vi "Read configuration.vi"(8 "error in":errorcluster, 11 "ExampleSequencer editor node in":refnum<class "ExampleSequencer editor node.lvclass">) -> (0 "error out":errorcluster, 2 "configuration":refnum<class "NISE_CEF_serializable configuration.lvclass">, 3 "ExampleSequencer editor node out":refnum<class "ExampleSequencer editor node.lvclass">)   [LabVIEW 2017, in "ExampleSequencer editor node.lvclass"]
uses:
  ExampleSequencer editor node.lvclass
  <vilib>/NI/Configuration Framework/serializable configuration/NISE_CEF_serializable configuration.lvclass
  ExampleSequencer editor node.lvclass/ExampleSequencer editor node.ctl
  module/configuration/ExampleSequencer configuration.lvclass
  C:/Program Files (x86)/National Instruments/LabVIEW 2017/vi.lib/NI/Configuration Framework/serializable configuration/NISE_CEF_serializable configuration.lvclass
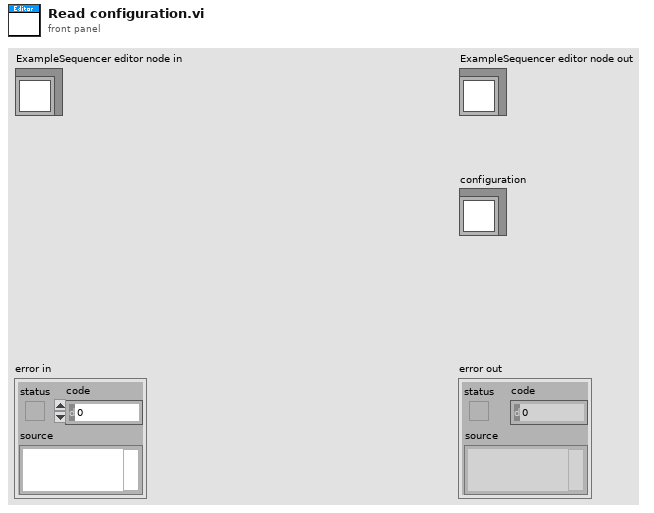
[diagram p1: front panel]
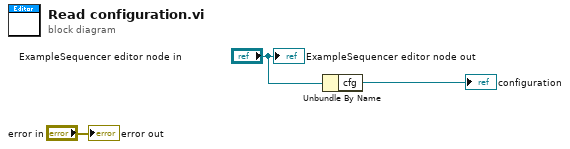
[diagram p0: block diagram]
diagram:
  n1 = Unbundle By Name("ExampleSequencer editor node in") -> ("cfg"=→"configuration":refnum<class "ExampleSequencer configuration.lvclass">)
  "error out" <- "error in"
  "ExampleSequencer editor node out" <- "ExampleSequencer editor node in"
